vi "Lines Filter-Annotation.vi"(7 "Annotation Seperator(#)":string="#", 8 "error in (no error)":errorcluster, 11 "Lines":string[](array[string])) -> (0 "error out":errorcluster, 3 "Config Text List":string[](array[string]))   [LabVIEW 2017, in "ini_configuration.lvlib"]
doc: "Removes the annotation lines, which start with Annotation Seperator(#), from a configuration file and trims the remaining lines."
uses:
  ini_configuration.lvlib
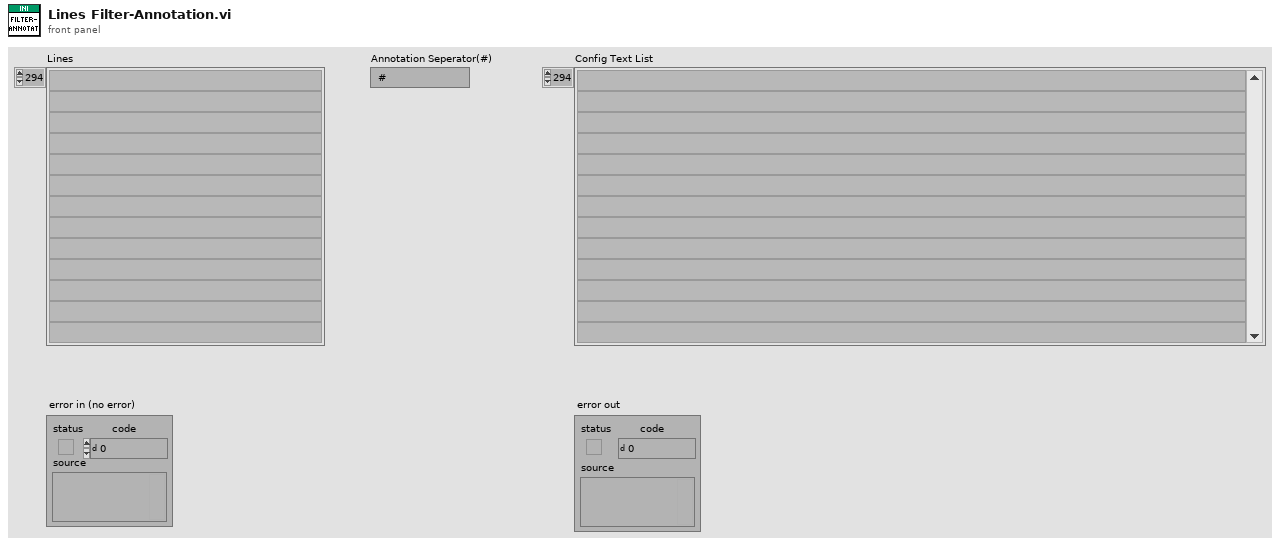
[diagram p1: front panel]
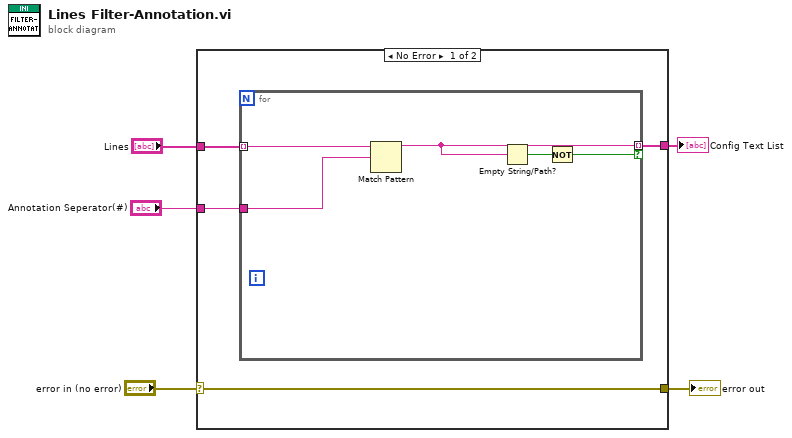
[diagram p0: block diagram]
diagram:
  n1 = case shown="No Error" "error in (no error)" {
    selector: "error in (no error)" -> [w7 w15]
    tunnel: [w7 w15] -> w4
    tunnel: "Lines" -> [w9 _]
    tunnel: [w8 _] -> w2
    tunnel: "Annotation Seperator(#)" -> [w6 _]
    frame No Error {
      n2 = for {
        tunnel: w9 -> [w13] mode=indexing
        tunnel: [w11] -> w8 mode=indexing if=w14
        tunnel: w6 -> [w10]
        n3 = Match Pattern(string=w13, regular expression=w10) -> (before substring=w11:string)  [unwired: 1 in, 3 out]
        n4 = Empty String/Path?(string/path=w11) -> (empty?=w12:bool)
        n5 = Not(x=w12) -> (.not. x?=w14:bool)
      }
    }
    frame Error {
    }
  }
  "error out" <- w4
  "Config Text List" <- w2
